vi "RT Loop - Acquisition and Logging V1-Config V2.vi"(8 "error in (no error)":errorcluster, 9 "Acquisition Data v1":T1={"Data Rate"=1, "Samples per Read"=0, "Number of Reads to Save"=0, "Data File Name"="", "TDMS Properties"=[], "Number of Channels"=4, "Channel Scale Array"=[0.0, 0.0, 0.0, 0.0, 0.0, 0.0, 0.0, 0.0, 0.0, 0.0, 0.0, 0.0, 0.0, 0.0, 0.0, 0.0, 0.0, 0.0, 0.0, 0.0, 0.0, 0.0, 0.0, 0.0], "Channel Names"=[], "Trigger - RMS Value"=0.0, "Trigger - Channel"=0, "Trigger - Time (Minute)"=0, "Input Configuration Array"=[]} {"Input Configuration Array" items=["AC Coupled", "DC Coupled", "IEPE AC Coupled"]; "Data Rate" items=["51.200 kS/s (NI 9234)"=1, "25.600 kS/s (NI 9234)"=2, "17.067 kS/s (NI 9234)"=3, "12.800 kS/s (NI 9234)"=4, "10.240 kS/s (NI 9234)"=5, "8.533 kS/s (NI 9234)"=6, "7.314 kS/s (NI 9234)"=7, "6.400 kS/s (NI 9234)"=8, "5.689 kS/s (NI 9234)"=9, "5.120 kS/s (NI 9234)"=10, "4.654 kS/s (NI 9234)"=11, "4.267 kS/s (NI 9234)"=12, "3.938 kS/s (NI 9234)"=13, "3.657 kS/s (NI 9234)"=14, "3.413 kS/s (NI 9234)"=15, "3.200 kS/s (NI 9234)"=16, "3.012 kS/s (NI 9234)"=17, "2.845 kS/s (NI 9234)"=18, "2.695 kS/s (NI 9234)"=19, "2.560 kS/s (NI 9234)"=20, "2.438 kS/s (NI 9234)"=21, "2.328 kS/s (NI 9234)"=22, "2.226 kS/s (NI 9234)"=23, "2.133 kS/s (NI 9234)"=24, "2.048 kS/s (NI 9234)"=25, "1.969 kS/s (NI 9234)"=26, "1.896 kS/s (NI 9234)"=27, "1.829 kS/s (NI 9234)"=28, "1.765 kS/s (NI 9234)"=29, "1.707 kS/s (NI 9234)"=30, "1.652 kS/s (NI 9234)"=31]}, 10 "Acquisition and Logging Queue":refnum<queue>, 11 "Message Queue":refnum<queue>) -> ()   [LabVIEW 2015]
uses:
  support/Message Queue/Message Cluster.ctl
  controls/Acquisition and Logging Configuration_v1.ctl
  <vilib>/LabVIEW Targets/FPGA/cRIO/shared/nicrio_ModuleControls/nicrio_cRIO-9234_DataRatesRing2.ctl
  controls/TDMS Properties.ctl
  <vilib>/LabVIEW Targets/FPGA/cRIO/shared/nicrio_ModuleControls/nicrio_cRIO-9234_ConfigModeRing.ctl
  controls/FPGA VI Reference.ctl
  Globals/Global - Configuration Options.vi
  Globals/Global - Monitoring Variables.vi
  support/Message Queue/Message Queue.lvlib
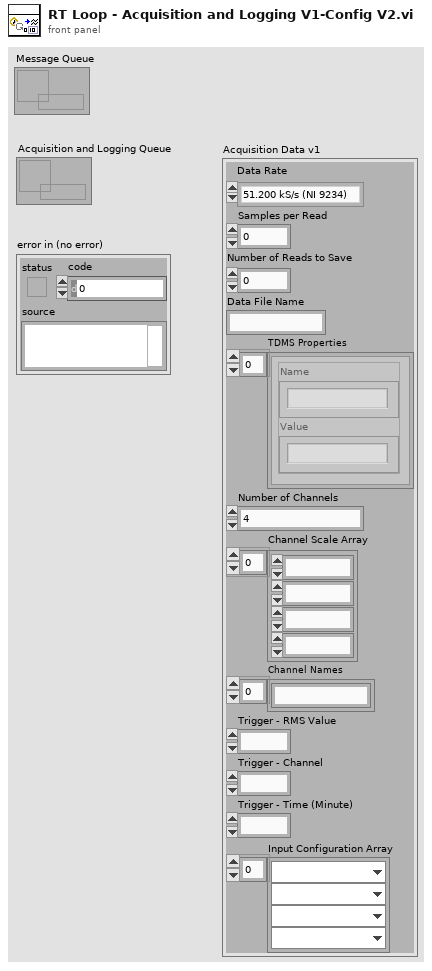
[diagram p1: front panel]
types:
  T1 = typedef "Acquisition and Logging Configuration_v1.ctl" = cluster{"Data Rate":T2, "Samples per Read":i32, "Number of Reads to Save":i32, "Data File Name":string, "TDMS Properties":T3[], "Number of Channels":i32, "Channel Scale Array":fxp<+,24,12>[], "Channel Names":string[], "Trigger - RMS Value":dbl, "Trigger - Channel":i32, "Trigger - Time (Minute)":i32, "Input Configuration Array":T4[]}
  T2 = typedef "nicrio_cRIO-9234_DataRatesRing2.ctl" = u8
  T3 = typedef "TDMS Properties.ctl" = cluster{"Name":string, "Value":string}
  T4 = typedef "nicrio_cRIO-9234_ConfigModeRing.ctl" = u8
  T5 = typedef "FPGA VI Reference.ctl" = refnum<k20>
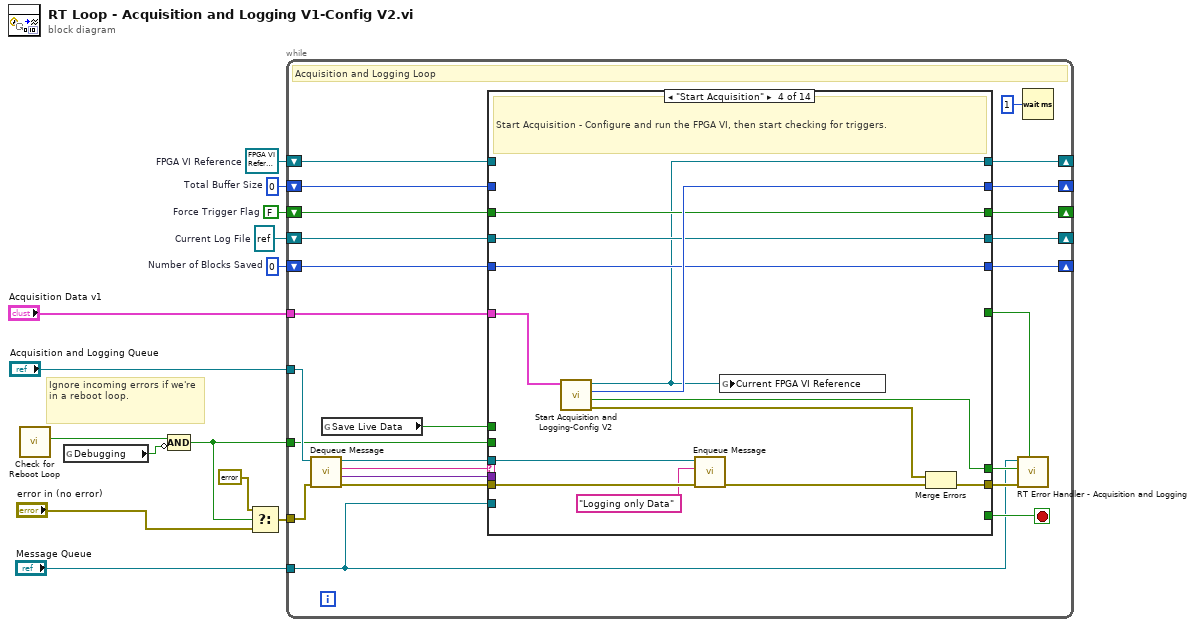
[diagram p0: block diagram]
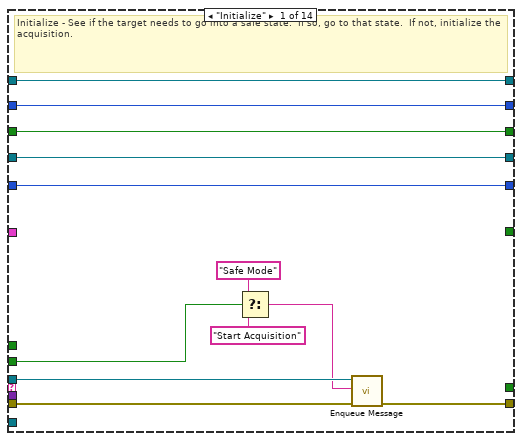
[diagram p2: hidden frame]
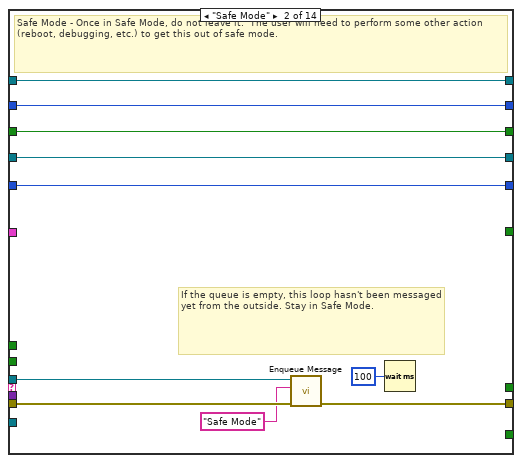
[diagram p3: hidden frame]
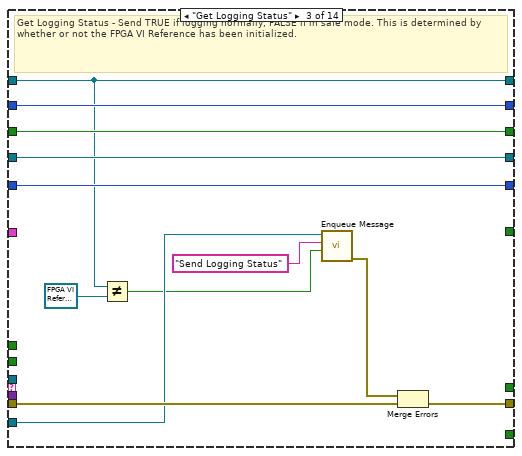
[diagram p4: hidden frame]
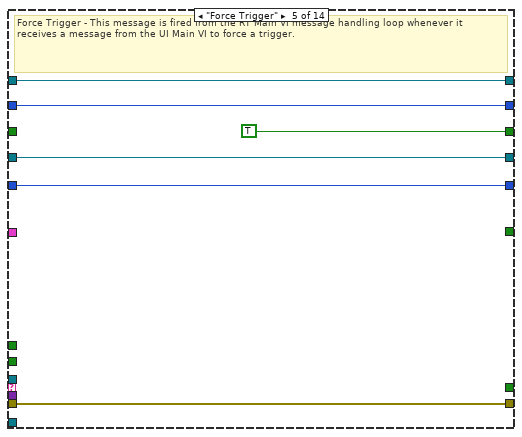
[diagram p5: hidden frame]
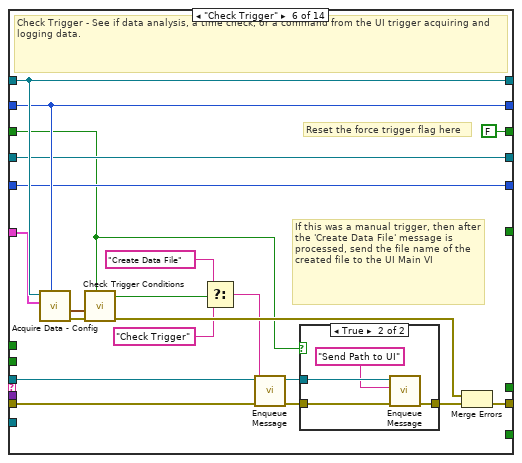
[diagram p6: hidden frame]
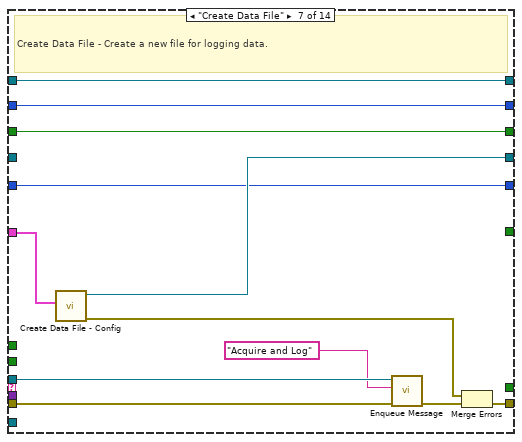
[diagram p8: hidden frame]
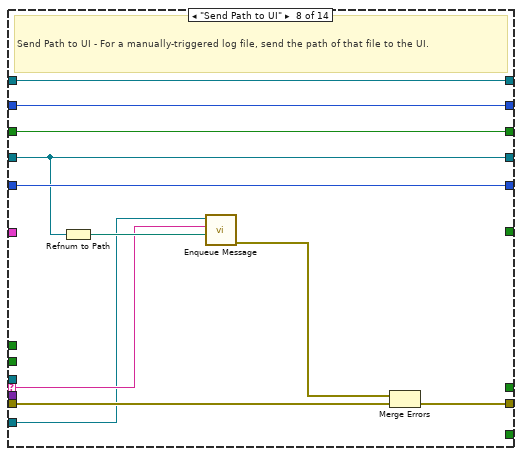
[diagram p9: hidden frame]
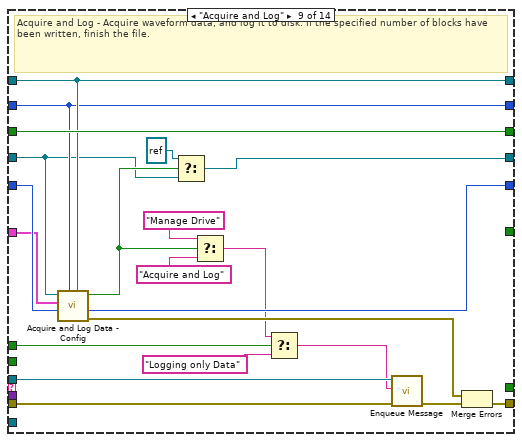
[diagram p10: hidden frame]
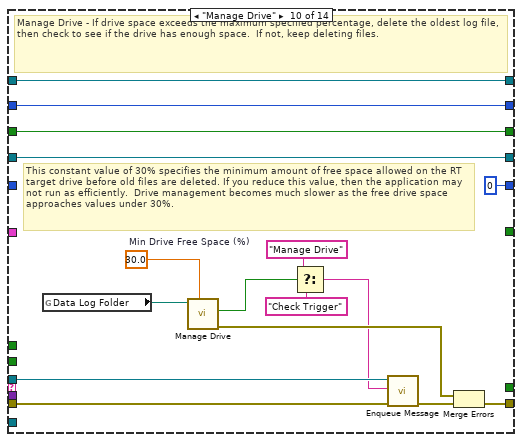
[diagram p11: hidden frame]
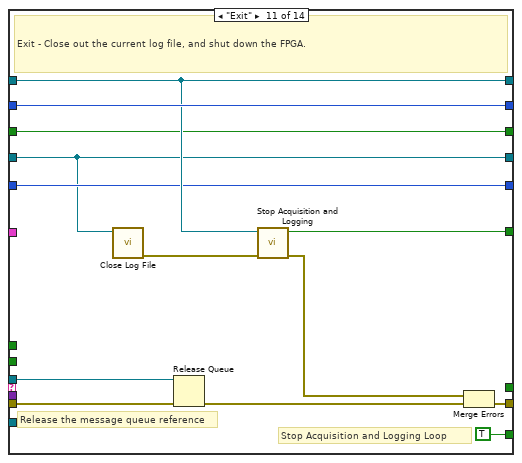
[diagram p12: hidden frame]
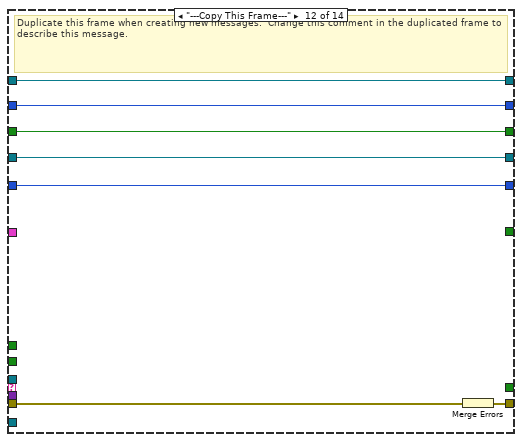
[diagram p13: hidden frame]
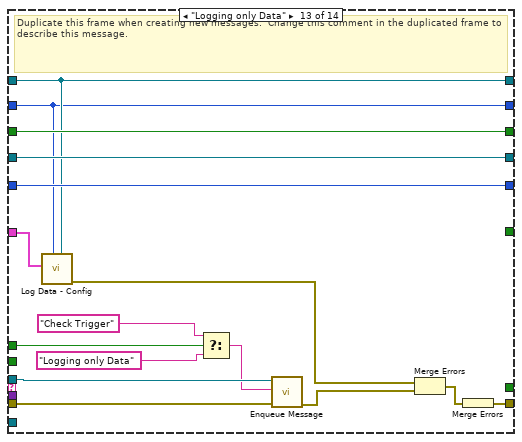
[diagram p14: hidden frame]
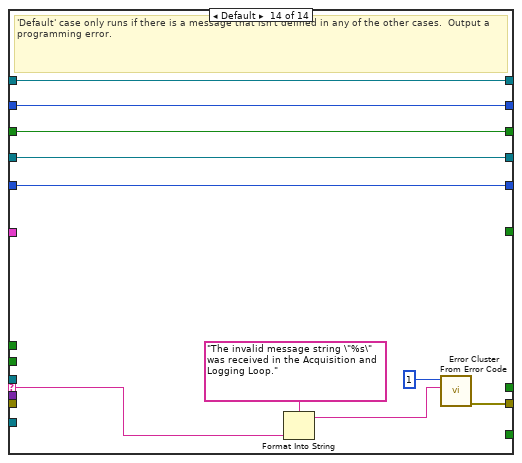
[diagram p15: hidden frame]
diagram:
  w8 = 0  # Number of Blocks Saved
  w9 = refnum<k34> refnum  # Current Log File
  w10 = FALSE  # Force Trigger Flag
  w11 = 0  # Total Buffer Size
  w12 = T5 refnum  # FPGA VI Reference
  # "Ignore incoming errors if we're in a reboot loop."
  n1 = call "Check for Reboot Loop.vi"() -> ("Start in Safe Mode?"=w4:bool)  [unwired: 10 in, 1 out]
  n2 = global read "Global - Configuration Options.vi" "Debugging"() -> (w3:bool)
  n3 = Compound Arithmetic op=AND(w4, invert w3) -> (w2:bool)
  n4 = Select(t=errorcluster {"status"=FALSE, "code"=0, "source"=""}, s=w2, f="error in (no error)") -> (s? t:f=w6:errorcluster)
  n5 = while {
    tunnel: "Acquisition and Logging Queue" -> [w35]
    tunnel: "Message Queue" -> [w19]
    shift-right: [w30] -> _
    shift-left: w12 -> [w32]
    shift-right: [w29] -> _
    shift-left: w11 -> [w31]
    tunnel: "Acquisition Data v1" -> [w28]
    shift-right: [w24] -> _
    shift-left: w10 -> [w25]
    shift-right: [w22] -> _
    shift-left: w9 -> [w23]
    shift-right: [w20] -> _
    shift-left: w8 -> [w21]
    tunnel: w6 -> [w17]
    tunnel: w2 -> [w16]
    stop <- w39 stop-if-true
    # "Acquisition and Logging Loop"
    n6 = call "Dequeue Message.vi"("error in (no error)"=w17, "Message Queue"=w35) -> ("error out"=w38:errorcluster, "Message Data"=w36:variant, "Message"=w37:string, "dup Message Queue"=w33:refnum<queue>)  [unwired: 6 in]
    n7 = global read "Global - Monitoring Variables.vi" "Save Live Data"() -> (w15:bool)
    n8 = case "Message Cases" shown="\"Start Acquisition\"" w37 {
      selector: w37 -> [_ _ _ _ _ _ _ w133 _ _ _ _ _ w222]
      tunnel: w33 -> [w48 w58 _ w80 _ w105 w124 _ w158 w170 w190 _ w209 _]
      tunnel: w38 -> [w49 w59 w73 w86 w92 w111 w128 w140 w161 w177 w186 w197 w206 _]
      tunnel: [w41 w57 w65 w85 w92 w110 w127 w131 w160 w173 w187 w196 w213 w220] -> w34
      tunnel: [_ _ _ _ _ _ _ _ _ _ TRUE _ _ _] -> w39
      tunnel: w36 -> [_ _ _ _ _ _ _ _ _ _ _ _ _ _]
      tunnel: w32 -> [w51 w61 w68 _ w91 w112 w129 w139 w153 w176 w184 w195 w204 w218]
      tunnel: w31 -> [w50 w60 w72 _ w90 w109 w126 w138 w152 w175 w185 w194 w203 w217]
      tunnel: [w51 w61 w68 w75 w91 w112 w129 w139 w153 w176 w184 w195 w204 w218] -> w30
      tunnel: [w50 w60 w72 w82 w90 w109 w126 w138 w152 w175 w185 w194 w203 w217] -> w29
      tunnel: w28 -> [_ _ _ w74 _ w93 w118 _ w141 _ _ _ w198 _]
      tunnel: [_ _ _ w83 _ _ _ _ _ _ _ _ _ _] -> w26
      tunnel: w25 -> [w44 w56 w71 w78 _ w94 w122 w137 w157 w163 w182 w193 w212 w216]
      tunnel: [w44 w56 w71 w78 TRUE ("Force Trigger Flag") FALSE ("Force Trigger Flag") w122 w137 w157 w163 w182 w193 w212 w216] -> w24
      tunnel: w23 -> [w43 w55 w70 w77 w89 w100 _ w135 w148 w174 w179 w192 w211 w215]
      tunnel: [w43 w55 w70 w77 w89 w100 w120 w135 w147 w174 w179 w192 w211 w215] -> w22
      tunnel: w21 -> [w42 w54 w69 w76 w87 w99 w119 w136 w151 _ w181 w191 w210 w214]
      tunnel: [w42 w54 w69 w76 w87 w99 w119 w136 w150 0 ("Number of Blocks Saved") w181 w191 w210 w214] -> w20
      tunnel: w19 -> [_ _ w66 _ _ _ _ w132 _ _ _ _ _ _]
      tunnel: [_ _ _ _ _ _ _ _ _ _ w178 _ _ _] -> w18
      tunnel: w16 -> [w40 _ _ _ _ _ _ _ _ _ _ _ _ _]
      tunnel: w15 -> [_ _ _ _ _ _ _ _ w145 _ _ _ w200 _]
      frame "Initialize" {
        # "Initialize - See if the target needs to go into a safe state.  If so, go to that state.  If not, initialize the acquisition."
        n9 = Select(t="Safe Mode", s=w40, f="Start Acquisition") -> (s? t:f=w45:string)
        n10 = call "Enqueue Message.vi"("error in (no error)"=w49, "Message"=w45, "Message Queue"=w48) -> ("error out"=w41:errorcluster)  [unwired: 7 in, 1 out]
      }
      frame "Safe Mode" {
        # "If the queue is empty, this loop hasn't been messaged yet from the outside. Stay in Safe Mode."
        # "Safe Mode - Once in Safe Mode, do not leave it.  The user will need to perform some other action (reboot, debugging, etc.) to get this out of safe mode."
        n11 = call "Enqueue Message.vi"("error in (no error)"=w59, "Message"="Safe Mode", "Message Queue"=w58) -> ("error out"=w57:errorcluster)  [unwired: 7 in, 1 out]
        n12 = Wait (ms)(milliseconds to wait=u32 100) -> ()  [unwired: 1 out]
      }
      frame "Get Logging Status" {
        # "Get Logging Status - Send TRUE if logging normally, FALSE if in safe mode. This is determined by whether or not the FPGA VI Reference has been initialized."
        n13 = Not Equal?(x=w68, y=T5 refnum ("FPGA VI Reference")) -> (x != y?=w63:bool)
        n14 = call "Enqueue Message.vi"("Message Data"=w63, "Message"="Send Logging Status", "Message Queue"=w66) -> ("error out"=w64:errorcluster)  [unwired: 7 in, 1 out]
        n15 = Merge Errors(w64, w73) -> (w65:errorcluster)
      }
      frame "Start Acquisition" {
        # "Start Acquisition - Configure and run the FPGA VI, then start checking for triggers."
        n16 = call "Start Acquisition and Logging-Config V2.vi"("Acquisition Data v1"=w74) -> ("FPGA VI Reference Out"=w75:T5, "Total Buffer Size"=w82:i32, "Wait on IRQ Timeout?"=w83:bool, "error out"=w84:errorcluster)  [unwired: 6 in]
        n17 = call "Enqueue Message.vi"("error in (no error)"=w86, "Message"="Logging only Data", "Message Queue"=w80) -> ("error out"=w81:errorcluster)  [unwired: 7 in, 1 out]
        n18 = global write "Global - Monitoring Variables.vi" "Current FPGA VI Reference"(w75) -> ()
        n19 = Merge Errors(w84, w81) -> (w85:errorcluster)
      }
      frame "Force Trigger" {
        # "Force Trigger - This message is fired from the RT Main VI message handling loop whenever it receives a message from the UI Main VI to force a trigger."
      }
      frame "Check Trigger" {
        # "If this was a manual trigger, then after the 'Create Data File' message is processed, send the file name of the created file to the UI Main VI"
        # "Reset the force trigger flag here"
        # "Check Trigger - See if data analysis, a time check, or a command from the UI trigger acquiring and logging data."
        n20 = call "Acquire Data - Config.vi"("Total Buffer Size"=w109, "Acquisition Data v1"=w93, "FPGA VI Reference"=w112) -> ("error out"=w107:errorcluster, "Waveform Data"=w106:waveform(sgl)[])  [unwired: 7 in]
        n21 = call "Check Trigger Conditions.vi"("Force Trigger?"=w94, "error in (no error)"=w107, "Waveform Data"=w106) -> ("error out"=w108:errorcluster, "Trigger Condition Met?"=w104:bool)  [unwired: 7 in]
        n22 = Select(t="Create Data File", s=w104, f="Check Trigger") -> (s? t:f=w101:string)
        n23 = call "Enqueue Message.vi"("error in (no error)"=w111, "Message"=w101, "Message Queue"=w105) -> ("error out"=w97:errorcluster, "dup Message Queue"=w95:refnum<queue>)  [unwired: 7 in]
        n24 = case shown="True" w94 {
          tunnel: w97 -> [w113 w116]
          tunnel: [w113 w117] -> w96
          tunnel: w95 -> [_ w115]
          frame False {
          }
          frame True {
            n25 = call "Enqueue Message.vi"("error in (no error)"=w116, "Message"="Send Path to UI", "Message Queue"=w115) -> ("error out"=w117:errorcluster)  [unwired: 7 in, 1 out]
          }
        }
        n26 = Merge Errors(w108, w96) -> (w110:errorcluster)
      }
      frame "Create Data File" {
        # "Create Data File - Create a new file for logging data."
        n27 = call "Create Data File - Config.vi"("Acquisition Data v1"=w118) -> ("error out"=w121:errorcluster, "TDMS File Reference"=w120:refnum<k34>)  [unwired: 9 in]
        n28 = call "Enqueue Message.vi"("error in (no error)"=w128, "Message"="Acquire and Log", "Message Queue"=w124) -> ("error out"=w125:errorcluster)  [unwired: 7 in, 1 out]
        n29 = Merge Errors(w121, w125) -> (w127:errorcluster)
      }
      frame "Send Path to UI" {
        # "Send Path to UI - For a manually-triggered log file, send the path of that file to the UI."
        n30 = Refnum to Path(1:w135) -> (0:w134:path)
        n31 = call "Enqueue Message.vi"("Message Data"=w134, "Message"=w133, "Message Queue"=w132) -> ("error out"=w130:errorcluster)  [unwired: 7 in, 1 out]
        n32 = Merge Errors(w130, w140) -> (w131:errorcluster)
      }
      frame "Acquire and Log" {
        # "Acquire and Log - Acquire waveform data, and log it to disk. If the specified number of blocks have been written, finish the file."
        n33 = call "Acquire and Log Data - Config .vi"("FPGA VI Reference"=w153, "Total Buffer Size"=w152, "Number of Blocks Saved in"=w151, "Acquisition Data v1"=w141, "TDMS File Reference"=w148) -> ("error out"=w156:errorcluster, "Number of Blocks Saved out"=w150:i32, "Logging Complete?"=w149:bool)  [unwired: 4 in]
        n34 = Select(t=refnum<k34> refnum, s=w149, f=w148) -> (s? t:f=w147:refnum<k34>)
        n35 = Select(t="Manage Drive", s=w149, f="Acquire and Log") -> (s? t:f=w143:string)
        n36 = Select(t=w143, s=w145, f="Logging only Data") -> (s? t:f=w142:string)
        n37 = call "Enqueue Message.vi"("error in (no error)"=w161, "Message"=w142, "Message Queue"=w158) -> ("error out"=w159:errorcluster)  [unwired: 7 in, 1 out]
        n38 = Merge Errors(w156, w159) -> (w160:errorcluster)
      }
      frame "Manage Drive" {
        w172 = 30.0  # Min Drive Free Space (%)
        # "This constant value of 30% specifies the minimum amount of free space allowed on the RT target drive before old files are deleted. If you reduce this value, then the application may not run as efficiently.  Drive management becomes much slower as the free drive space approaches values under 30%."
        # "Manage Drive - If drive space exceeds the maximum specified percentage, delete the oldest log file, then check to see if the drive has enough space.  If not, keep deleting files."
        n39 = global read "Global - Configuration Options.vi" "Data Log Folder"() -> (w162:path)
        n40 = call "Manage Drive.vi"("Min Drive Free Space (%)"=w172, "Data Folder"=w162) -> ("error out"=w169:errorcluster, "Drive Space Below Limit"=w168:bool)  [unwired: 8 in]
        n41 = Select(t="Manage Drive", s=w168, f="Check Trigger") -> (s? t:f=w165:string)
        n42 = call "Enqueue Message.vi"("error in (no error)"=w177, "Message"=w165, "Message Queue"=w170) -> ("error out"=w171:errorcluster)  [unwired: 7 in, 1 out]
        n43 = Merge Errors(w169, w171) -> (w173:errorcluster)
      }
      frame "Exit" {
        # "Stop Acquisition and Logging Loop"
        # "Release the message queue reference"
        # "Exit - Close out the current log file, and shut down the FPGA."
        n44 = call "Close Log File.vi"("Log File"=w179) -> ("error out"=w180:errorcluster)  [unwired: 10 in]
        n45 = Release Queue(queue=w190, error in (no error)=w186) -> (error out=w188:errorcluster)  [unwired: 1 in, 2 out]
        n46 = call "Stop Acquisition and Logging.vi"("error in (no error)"=w180, "FPGA VI Reference"=w184) -> ("error out"=w183:errorcluster, "Stop FPGA Timeout?"=w178:bool)  [unwired: 8 in]
        n47 = Merge Errors(w183, w188) -> (w187:errorcluster)
      }
      frame "---Copy This Frame---" {
        # "Duplicate this frame when creating new messages.  Change this comment in the duplicated frame to describe this message."
        n48 = Merge Errors(w197) -> (w196:errorcluster)
      }
      frame "Logging only Data" {
        # "Duplicate this frame when creating new messages.  Change this comment in the duplicated frame to describe this message."
        n49 = call "Log Data - Config.vi"("FPGA VI Reference"=w204, "Total Buffer Size"=w203, "Acquisition Data v1"=w198) -> ("error out"=w205:errorcluster)  [unwired: 8 in]
        n50 = Select(t="Check Trigger" ("Message"), s=w200, f="Logging only Data" ("Message")) -> (s? t:f=w201:string)
        n51 = call "Enqueue Message.vi"("error in (no error)"=w206, "Message"=w201, "Message Queue"=w209) -> ("error out"=w208:errorcluster)  [unwired: 7 in, 1 out]
        n52 = Merge Errors(w205, w208) -> (w207:errorcluster)
        n53 = Merge Errors(w207) -> (w213:errorcluster)
      }
      frame Default {
        # "'Default' case only runs if there is a message that isn't defined in any of the other cases.  Output a programming error."
        n54 = Format Into String(format string="The invalid message string \"%s\" was received in the Acquisition and Logging Loop." ("Unknown Message Error Text"), w222) -> (resulting string=w219:string)  [unwired: 2 in, 1 out]
        n55 = call <vilib>:"Error Cluster From Error Code.vi"("error message (\"\")"=w219, "error code (0)"=1) -> ("error out"=w220:errorcluster)  [unwired: 7 in]
      }
    }
    n56 = call "RT Error Handler - Acquisition and Logging.vi"("Stop FPGA Timeout"=w18, "error in (no error)"=w34, "IRQ Timeout"=w26, "Message Queue"=w19) -> ()  [unwired: 7 in, 1 out]
    n57 = Wait (ms)(milliseconds to wait=u32 1) -> ()  [unwired: 1 out]
  }
